vi "FilterParamInitial.vi"(8 "Error In":errorcluster, 11 "FiltersParam":refnum<vi>) -> (0 "Error Out":errorcluster, 2 "FiltersParam Out":T1={"Kernel"=[[1.0, 1.0, 1.0], [1.0, 1.0, 1.0], [1.0, 1.0, 1.0]], "Kernel Size"=3, "Filter Size X"=0, "Filter Size Y"=0, "Tolerance %"=0, "Divider"=0.0, "FilterFunction"=enum."Smoothing - Low Pass", "Sigma"=0.0, "LThres"=0.0, "HThresh"=0.0, "Windows Size"=0} {"Kernel Size" min=3 max=7 step=2})   [LabVIEW 2015]
uses:
  Controls/FiltersParam_Type.ctl
  <vilib>/vision/NI_Vision_Development_Module.lvlib
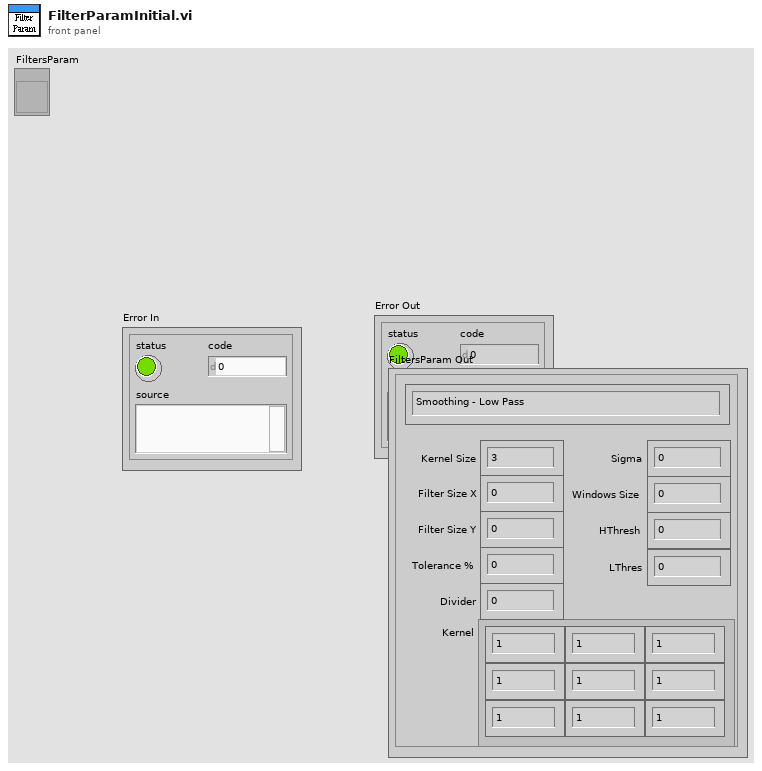
[diagram p1: front panel]
types:
  T1 = typedef "FiltersParam_Type.ctl" = cluster{"Kernel":sgl[][], "Kernel Size":i32, "Filter Size X":i32, "Filter Size Y":i32, "Tolerance %":i32, "Divider":sgl, "FilterFunction":enum16{"Smoothing - Low Pass", "Smoothing - Local Average", "Smoothing - Guassian", "Smoothing - Median", "------------------------------------", "Edge Detection - Laplacian", "Edge Detection - Diff", "Edge Detection - Prewitt", "Edge Detection - Sobel", "Edge Detection - Roberts", "Edge Detection - Canny", "Edge Detection - Gradient", "Edge Detection - Sigma", "----------------------------------------", "Convolution - Highlight Details", "Convolution - Custom"}, "Sigma":sgl, "LThres":sgl, "HThresh":sgl, "Windows Size":i32}
  T2 = enum16{"Smoothing - Low Pass", "Smoothing - Local Average", "Smoothing - Guassian", "Smoothing - Median", "------------------------------------", "Edge Detection - Laplacian", "Edge Detection - Diff", "Edge Detection - Prewitt", "Edge Detection - Sobel", "Edge Detection - Roberts", "Edge Detection - Canny", "Edge Detection - Gradient", "Edge Detection - Sigma", "----------------------------------------", "Convolution - Highlight Details", "Convolution - Custom"}
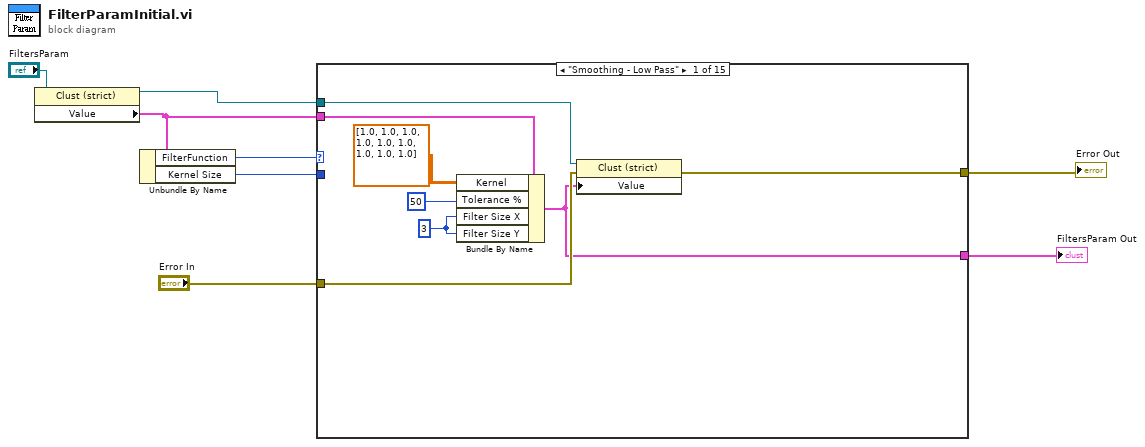
[diagram p0: block diagram]
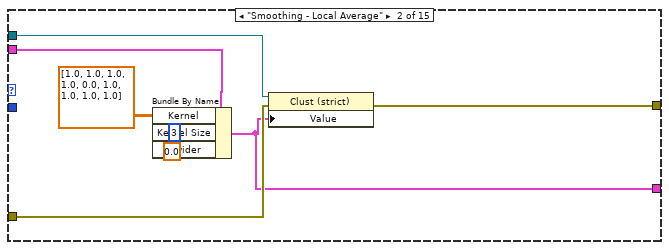
[diagram p2: hidden frame]
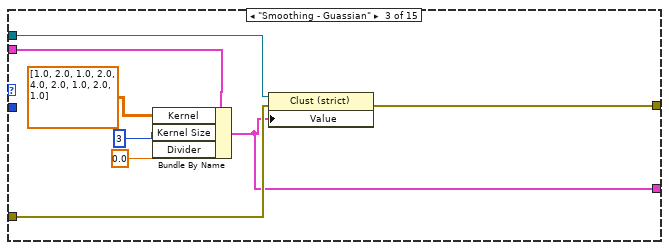
[diagram p3: hidden frame]
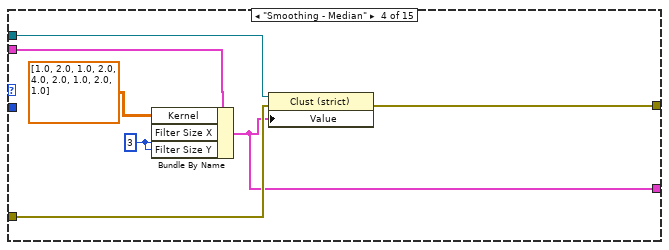
[diagram p4: hidden frame]
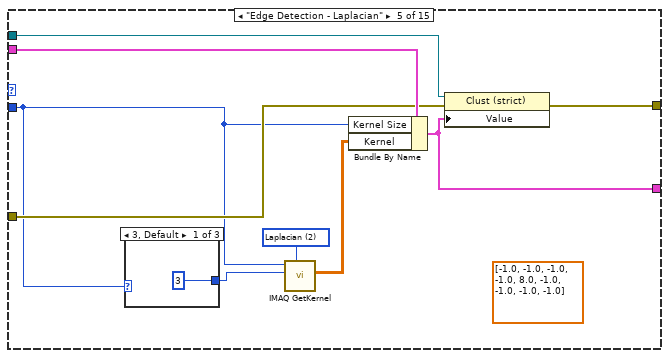
[diagram p5: hidden frame]
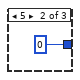
[diagram p6: hidden frame]
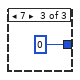
[diagram p7: hidden frame]
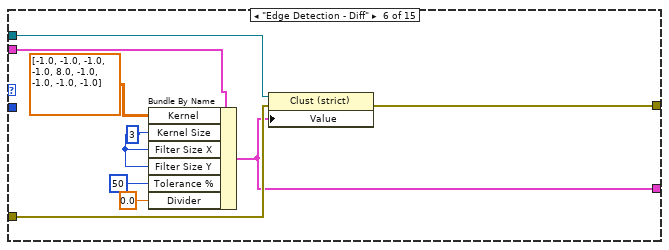
[diagram p8: hidden frame]
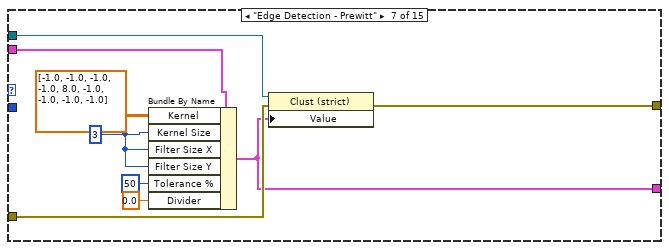
[diagram p9: hidden frame]
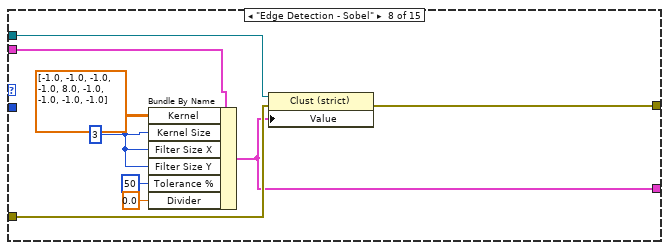
[diagram p10: hidden frame]
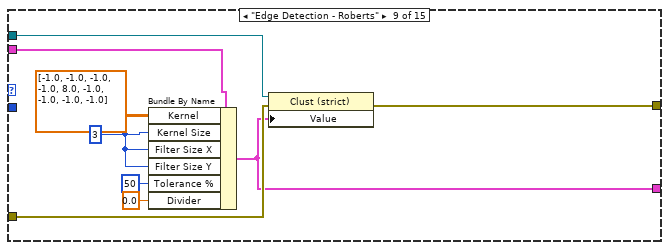
[diagram p11: hidden frame]
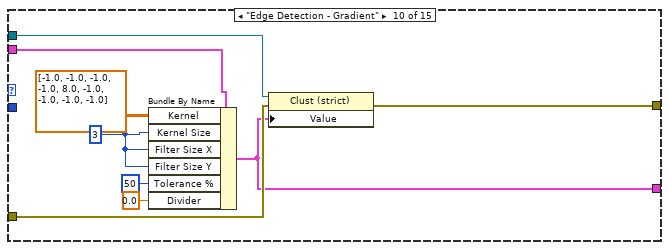
[diagram p12: hidden frame]
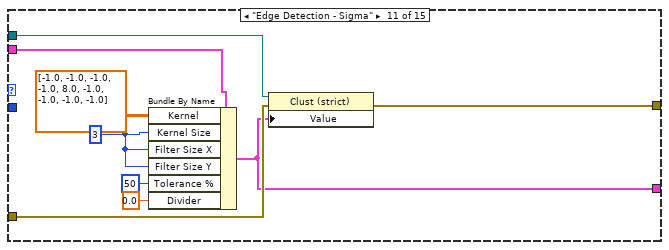
[diagram p13: hidden frame]
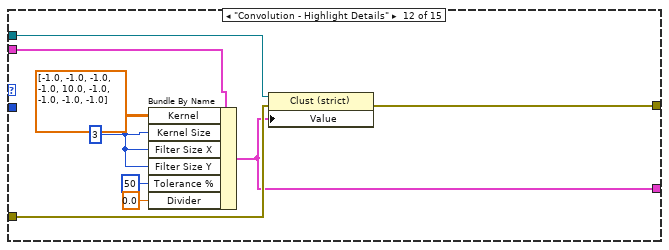
[diagram p14: hidden frame]
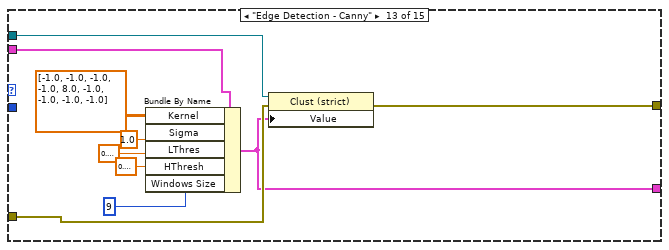
[diagram p15: hidden frame]
diagram:
  n1 = property class="Clust (strict)"(reference="FiltersParam") -> (reference out=w7:refnum<vi>, "Value"=w6:T1)  [unwired: 1 in, 1 out]
  n2 = Unbundle By Name(w6) -> ("FilterFunction"=w5:T2, "Kernel Size"=w2:i32)
  n3 = case shown="\"Smoothing - Low Pass\"" w5 {
    tunnel: w7 -> [w13 w23 w31 w38 w48 w59 w68 w77 w86 w95 w104 w113 w123 _ _]
    tunnel: w6 -> [w12 w20 w28 w37 w47 w58 w67 w76 w85 w94 w103 w112 w122 w125 w127]
    tunnel: "Error In" -> [w11 w19 w27 w35 w46 w54 w63 w72 w81 w90 w99 w108 w117 w126 w128]
    tunnel: [w10 w18 w26 w34 w45 w53 w62 w71 w80 w89 w98 w107 w116 w126 w128] -> w3
    tunnel: w2 -> [_ _ _ _ w42 _ _ _ _ _ _ _ _ _ _]
    tunnel: [w9 w17 w25 w33 w40 w52 w61 w70 w79 w88 w97 w106 w115 w125 w127] -> w1
    frame "Smoothing - Low Pass" {
      w14 = 3 ("Filter Size X")
      n4 = Bundle By Name(cluster=w12, "Kernel"=sgl[][] [[1.0, 1.0, 1.0], [1.0, 1.0, 1.0], [1.0, 1.0, 1.0]], "Tolerance %"=50, "Filter Size X"=w14, "Filter Size Y"=w14) -> (w9:T1)
      n5 = property class="Clust (strict)"(reference=w13, error in=w11, "Value"=w9) -> (error out=w10:errorcluster)  [unwired: 1 out]
    }
    frame "Smoothing - Local Average" {
      n6 = Bundle By Name(cluster=w20, "Kernel"=sgl[][] [[1.0, 1.0, 1.0], [1.0, 0.0, 1.0], [1.0, 1.0, 1.0]], "Kernel Size"=3, "Divider"=sgl 0.0) -> (w17:T1)
      n7 = property class="Clust (strict)"(reference=w23, error in=w19, "Value"=w17) -> (error out=w18:errorcluster)  [unwired: 1 out]
    }
    frame "Smoothing - Guassian" {
      n8 = Bundle By Name(cluster=w28, "Kernel"=sgl[][] [[1.0, 2.0, 1.0], [2.0, 4.0, 2.0], [1.0, 2.0, 1.0]], "Kernel Size"=3, "Divider"=sgl 0.0) -> (w25:T1)
      n9 = property class="Clust (strict)"(reference=w31, error in=w27, "Value"=w25) -> (error out=w26:errorcluster)  [unwired: 1 out]
    }
    frame "Smoothing - Median" {
      w36 = 3 ("Kernel Size")
      n10 = Bundle By Name(cluster=w37, "Kernel"=sgl[][] [[1.0, 2.0, 1.0], [2.0, 4.0, 2.0], [1.0, 2.0, 1.0]], "Filter Size X"=w36, "Filter Size Y"=w36) -> (w33:T1)
      n11 = property class="Clust (strict)"(reference=w38, error in=w35, "Value"=w33) -> (error out=w34:errorcluster)  [unwired: 1 out]
    }
    frame "Edge Detection - Laplacian" {
      w44 = u16 2 items=["Gradient"=1, "Laplacian"=2, "Smoothing"=3, "Gaussian"=4] ("Kernel Family")
      (unwired) sgl[][] [[-1.0, -1.0, -1.0], [-1.0, 8.0, -1.0], [-1.0, -1.0, -1.0]] ("Kernel")
      n12 = case shown="3, Default" w42 {
        tunnel: [3 ("Kernel Code") 0 ("Kernel Code") 0 ("Kernel Code")] -> w43
        frame 3, Default {
        }
        frame 5 {
        }
        frame 7 {
        }
      }
      n13 = call "IMAQ GetKernel"("Kernel Family"=w44, "Kernel Number"=w43, "Kernel Size (3,5,...)"=w42) -> ("Kernel"=w41:sgl[][])  [unwired: 5 in, 3 out]
      n14 = Bundle By Name(cluster=w47, "Kernel Size"=w42, "Kernel"=w41) -> (w40:T1)
      n15 = property class="Clust (strict)"(reference=w48, error in=w46, "Value"=w40) -> (error out=w45:errorcluster)  [unwired: 1 out]
    }
    frame "Edge Detection - Diff" {
      w55 = 3 ("Kernel Size")
      n16 = Bundle By Name(cluster=w58, "Kernel"=sgl[][] [[-1.0, -1.0, -1.0], [-1.0, 8.0, -1.0], [-1.0, -1.0, -1.0]], "Kernel Size"=w55, "Filter Size X"=w55, "Filter Size Y"=w55, "Tolerance %"=50, "Divider"=sgl 0.0) -> (w52:T1)
      n17 = property class="Clust (strict)"(reference=w59, error in=w54, "Value"=w52) -> (error out=w53:errorcluster)  [unwired: 1 out]
    }
    frame "Edge Detection - Prewitt" {
      w64 = 3 ("Kernel Size")
      n18 = Bundle By Name(cluster=w67, "Kernel"=sgl[][] [[-1.0, -1.0, -1.0], [-1.0, 8.0, -1.0], [-1.0, -1.0, -1.0]], "Kernel Size"=w64, "Filter Size X"=w64, "Filter Size Y"=w64, "Tolerance %"=50, "Divider"=sgl 0.0) -> (w61:T1)
      n19 = property class="Clust (strict)"(reference=w68, error in=w63, "Value"=w61) -> (error out=w62:errorcluster)  [unwired: 1 out]
    }
    frame "Edge Detection - Sobel" {
      w73 = 3 ("Kernel Size")
      n20 = Bundle By Name(cluster=w76, "Kernel"=sgl[][] [[-1.0, -1.0, -1.0], [-1.0, 8.0, -1.0], [-1.0, -1.0, -1.0]], "Kernel Size"=w73, "Filter Size X"=w73, "Filter Size Y"=w73, "Tolerance %"=50, "Divider"=sgl 0.0) -> (w70:T1)
      n21 = property class="Clust (strict)"(reference=w77, error in=w72, "Value"=w70) -> (error out=w71:errorcluster)  [unwired: 1 out]
    }
    frame "Edge Detection - Roberts" {
      w82 = 3 ("Kernel Size")
      n22 = Bundle By Name(cluster=w85, "Kernel"=sgl[][] [[-1.0, -1.0, -1.0], [-1.0, 8.0, -1.0], [-1.0, -1.0, -1.0]], "Kernel Size"=w82, "Filter Size X"=w82, "Filter Size Y"=w82, "Tolerance %"=50, "Divider"=sgl 0.0) -> (w79:T1)
      n23 = property class="Clust (strict)"(reference=w86, error in=w81, "Value"=w79) -> (error out=w80:errorcluster)  [unwired: 1 out]
    }
    frame "Edge Detection - Gradient" {
      w91 = 3 ("Kernel Size")
      n24 = Bundle By Name(cluster=w94, "Kernel"=sgl[][] [[-1.0, -1.0, -1.0], [-1.0, 8.0, -1.0], [-1.0, -1.0, -1.0]], "Kernel Size"=w91, "Filter Size X"=w91, "Filter Size Y"=w91, "Tolerance %"=50, "Divider"=sgl 0.0) -> (w88:T1)
      n25 = property class="Clust (strict)"(reference=w95, error in=w90, "Value"=w88) -> (error out=w89:errorcluster)  [unwired: 1 out]
    }
    frame "Edge Detection - Sigma" {
      w100 = 3 ("Kernel Size")
      n26 = Bundle By Name(cluster=w103, "Kernel"=sgl[][] [[-1.0, -1.0, -1.0], [-1.0, 8.0, -1.0], [-1.0, -1.0, -1.0]], "Kernel Size"=w100, "Filter Size X"=w100, "Filter Size Y"=w100, "Tolerance %"=50, "Divider"=sgl 0.0) -> (w97:T1)
      n27 = property class="Clust (strict)"(reference=w104, error in=w99, "Value"=w97) -> (error out=w98:errorcluster)  [unwired: 1 out]
    }
    frame "Convolution - Highlight Details" {
      w109 = 3 ("Kernel Size")
      n28 = Bundle By Name(cluster=w112, "Kernel"=sgl[][] [[-1.0, -1.0, -1.0], [-1.0, 10.0, -1.0], [-1.0, -1.0, -1.0]], "Kernel Size"=w109, "Filter Size X"=w109, "Filter Size Y"=w109, "Tolerance %"=50, "Divider"=sgl 0.0) -> (w106:T1)
      n29 = property class="Clust (strict)"(reference=w113, error in=w108, "Value"=w106) -> (error out=w107:errorcluster)  [unwired: 1 out]
    }
    frame "Edge Detection - Canny" {
      n30 = Bundle By Name(cluster=w122, "Kernel"=sgl[][] [[-1.0, -1.0, -1.0], [-1.0, 8.0, -1.0], [-1.0, -1.0, -1.0]], "Sigma"=sgl 1.0, "LThres"=sgl 0.2, "HThresh"=sgl 0.7, "Windows Size"=9) -> (w115:T1)
      n31 = property class="Clust (strict)"(reference=w123, error in=w117, "Value"=w115) -> (error out=w116:errorcluster)  [unwired: 1 out]
    }
    frame "------------------------------------", Default {
    }
    frame "----------------------------------------" {
    }
  }
  "Error Out" <- w3
  "FiltersParam Out" <- w1
